vi "GL Position.vi"(5 "Wait for Motion Complete":bool=TRUE, 6 "error in (no error)":errorcluster, 8 "Axis":T1 items=["Axis 1", "Axis 2", "Axis 3", "Axis 4", "Axis 5", "Axis 6", "Axis 7", "Axis 8"], 9 "Galil.IGalil":refnum<k7>) -> (0 "error out":errorcluster, 2 "Axis Out":T1 items=["Axis 1", "Axis 2", "Axis 3", "Axis 4", "Axis 5", "Axis 6", "Axis 7", "Axis 8"], 3 "ref out":refnum<k7>, 4 "Axis Position":i32)   [LabVIEW 2022 SP3]
doc: "Sets the operation mode for an axis or vector space."
uses:
  GL Axis Control.ctl
  Command Menu.ctl
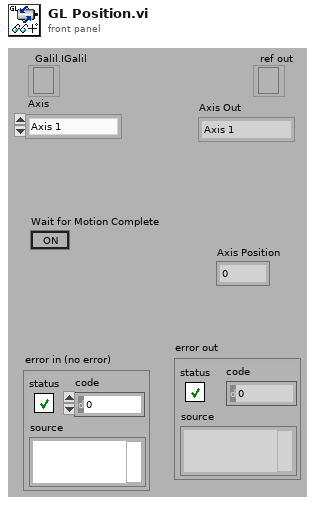
[diagram p1: front panel]
types:
  T1 = typedef "GL Axis Control.ctl" = u16
  T2 = typedef "Command Menu.ctl" = enum16{"CommandPassThrough", "Abort Motion", "Define Pos", "Velocity", "Acceleration", "Deceleration", "Position Rel", "Postion Abs", "Begin Move", "After Move", "Home", "KI", "KD", "KP", "IL", "Config I/O", "Set Bit", "Clear Bit", "Motor Off", "Moto On", "Status", "Execute", "Halt Execute", "HX Status", "Tell Velocity", "Check Motion", "BreakPoint", "Tell Position", "Current Code Line", "Tell Switches", "OC Force On", "OC Off", "Pos Soft Limit", "Rev Soft Limit"}
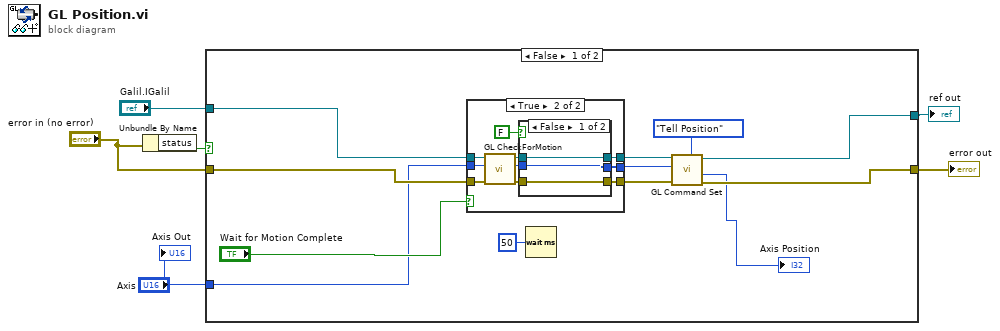
[diagram p0: block diagram]
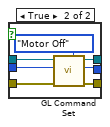
[diagram p3: hidden frame]
diagram:
  n1 = Unbundle By Name("error in (no error)") -> ("status"=w4:bool)
  n2 = case shown="False" w4 {
    tunnel: "error in (no error)" -> [w17 w43]
    tunnel: [w18 w43] -> w5
    tunnel: "Axis" -> [w9 _]
    tunnel: [w15 w42] -> w2
    tunnel: "Galil.IGalil" -> [w14 w42]
    frame False {
      n3 = case shown="True" "Wait for Motion Complete" {
        tunnel: [w21 w25] -> w12
        tunnel: [w20 w26] -> w11
        tunnel: w14 -> [w21 w31]
        tunnel: w9 -> [w19 w30]
        tunnel: w17 -> [w20 w29]
        tunnel: [w19 w23] -> w7
        frame False {
        }
        frame True {
          n4 = call "GL CheckForMotion.vi"("error in"=w29, "Axis"=w30, "Refnum in"=w31) -> ("error out"=w27:errorcluster, "Axis out"=w24:T1, "Refnum out"=w28:refnum<k7>)  [unwired: 6 in]
          n5 = case shown="False" FALSE {
            tunnel: w28 -> [w34 w41]
            tunnel: w27 -> [w33 w40]
            tunnel: [w33 w39] -> w26
            tunnel: [w34 w38] -> w25
            tunnel: w24 -> [w32 w36]
            tunnel: [w32 w35] -> w23
            frame False {
            }
            frame True {
              n6 = call "GL Command Set.vi"("Command"=Command_Menu."Motor Off", "error in (no error)"=w40, "Axis"=w36, "Galil.IGalil"=w41) -> ("error out"=w39:errorcluster, "Axis Out"=w35:T1, "ref out"=w38:refnum<k7>)  [unwired: 3 in, 2 out]
            }
          }
        }
      }
      n7 = Wait (ms)(milliseconds to wait=u32 50) -> ()  [unwired: 1 out]
      n8 = call "GL Command Set.vi"("Command"=Command_Menu."Tell Position", "error in (no error)"=w11, "Axis"=w7, "Galil.IGalil"=w12) -> ("error out"=w18:errorcluster, "Response#"=→"Axis Position":i32, "ref out"=w15:refnum<k7>)  [unwired: 3 in, 2 out]
    }
    frame True {
    }
  }
  "error out" <- w5
  "ref out" <- w2
  "Axis Out" <- "Axis"
